vi "Image_Crop_Fixed_Area_old.vi"(8 "Particle Measurements":dbl[][](array[numeric]), 9 "Image":T1, 11 "Object size threshold":dbl=500.0) -> (0 "Object detected":bool, 3 "output array":i32[](array[numeric]))   [LabVIEW 2019]
uses:
  <vilib>/vision/Image Controls.llb/IMAQ Image.ctl
panel:
  out "error out":errorcluster={"status"=TRUE, "code"=-1074396120, "source"="IMAQ Get Image Size\n  "}
  out "Image size/2":dbl
  out "Max x":dbl
  out "Max y":dbl
  in  "Image Border":dbl=20.0
  out "Max area detected":dbl
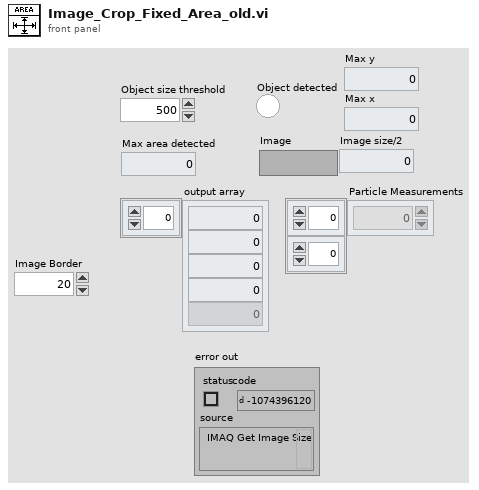
[diagram p1: front panel]
types:
  T1 = typedef "IMAQ Image.ctl" = refnum<image>
  T2 = cluster{"Global Rectangle":i32[], "Contours":cluster{"ID":enum32{"External", "Internal"}, "Type":u32, "Coordinates":i32[]}[]}
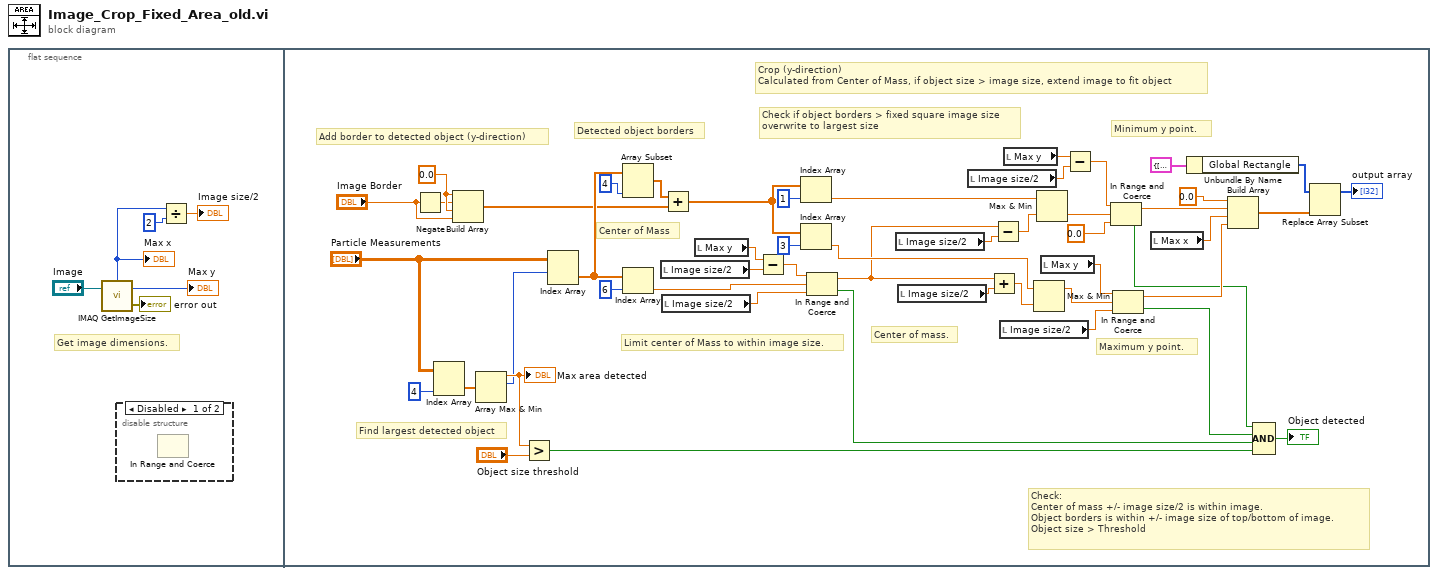
[diagram p0: block diagram]
diagram:
  n1 = flat-sequence {
    frame #0 {
      # "Get image dimensions."
      n2 = call "IMAQ GetImageSize"("Image"="Image") -> ("Y Resolution"=→"Max y":i32, "X Resolution"=w4:i32, "error out"=→"error out":errorcluster)  [unwired: 3 in]
      "Max x" <- w4
      n3 = disable-structure shown="Disabled" {
        frame Disabled {
          n4 = In Range and Coerce() -> ()  [unwired: 3 in, 2 out]
        }
        frame Enabled {
        }
      }
      n5 = Divide(x=w4, y=2) -> (x/y=→"Image size/2":dbl)
    }
    frame #1 {
      w39 = 0.0 ("element")
      # "Check:\nCenter of mass +/- image size/2 is within image.\nObject borders is within +/- image size of top/bottom of image.\nObject size > Threshold"
      # "Maximum y point."
      # "Minimum y point."
      # "Center of mass."
      # "Limit center of Mass to within image size."
      # "Add border to detected object (y-direction)"
      # "Find largest detected object"
      # "Check if object borders > fixed square image size\noverwrite to largest size"
      # "Detected object borders"
      # "Center of Mass"
      # "Crop (y-direction)\nCalculated from Center of Mass, if object size > image size, extend image to fit object"
      n6 = Negate(x="Image Border") -> (-x=w37:dbl)
      n7 = Index Array(array="Particle Measurements", index (col)=4 ("index (row)")) -> (element=w52:dbl[])  [unwired: 1 in]
      n8 = Build Array(w39, w37, w39, "Image Border") -> (w36:dbl[])
      n9 = Array Max & Min(array=w52) -> (max value=w50:dbl, max index (indices)=w47:i32)  [unwired: 2 out]
      "Max area detected" <- w50
      n10 = Greater?(x=w50, y="Object size threshold") -> (0:w49:bool)
      n11 = Index Array(array="Particle Measurements", index (row)=w47) -> (element=w46:dbl[])  [unwired: 1 in]
      n12 = Array Subset(array=w46, length=4) -> (w44:dbl[])  [unwired: 1 in]
      n13 = Index Array(array=w46, index=6) -> (element=w24:dbl)
      n14 = local read "Image size/2"() -> (w30:dbl)
      n15 = local read "Image size/2"() -> (w22:dbl)
      n16 = Add(x=w44, y=w36) -> (x+y=w27:dbl[])
      n17 = local read "Max y"() -> (w31:dbl)
      n18 = Subtract(x=w31, y=w30) -> (x-y=w23:dbl)
      n19 = Index Array(array=w27, index=1) -> (element=w42:dbl)
      n20 = Index Array(array=w27, index=3) -> (element=w40:dbl)
      n21 = In Range and Coerce(upper limit=w23, x=w24, lower limit=w22) -> (coerced(x)=w20:dbl, In Range?=w21:bool)
      n22 = local read "Image size/2"() -> (w26:dbl)
      n23 = local read "Image size/2"() -> (w25:dbl)
      n24 = local read "Image size/2"() -> (w15:dbl)
      n25 = Add(x=w20, y=w25) -> (x+y=w29:dbl)
      n26 = Subtract(x=w20, y=w26) -> (x-y=w28:dbl)
      n27 = local read "Image size/2"() -> (w12:dbl)
      n28 = local read "Max y"() -> (w16:dbl)
      n29 = Max & Min(x=w40, y=w29) -> (max(x,y)=w7:dbl)  [unwired: 1 out]
      n30 = Max & Min(x=w42, y=w28) -> (min(x,y)=w19:dbl)  [unwired: 1 out]
      n31 = local read "Max y"() -> (w13:dbl)
      n32 = Subtract(x=w16, y=w15) -> (x-y=w14:dbl)
      n33 = In Range and Coerce(upper limit=w14, x=w19, lower limit=0.0 ("x")) -> (coerced(x)=w17:dbl, In Range?=w9:bool)
      n34 = In Range and Coerce(upper limit=w13, x=w7, lower limit=w12) -> (coerced(x)=w11:dbl, In Range?=w10:bool)
      n35 = local read "Max x"() -> (w32:dbl)
      n36 = Unbundle By Name(T2 {"Global Rectangle"=[106, 29, 356, 265], "Contours"=[{"ID"=enum."External", "Type"=3, "Coordinates"=[106, 29, 356, 265]}]} ("Crop to object")) -> ("Global Rectangle"=w55:i32[])
      n37 = Build Array(0.0 ("x"), w17, w32, w11) -> (w35:dbl[])
      n38 = Compound Arithmetic op=AND(w9, w10, w21, w49) -> (→"Object detected":bool)
      n39 = Replace Array Subset(array=w55, new element=w35) -> (→"output array":i32[])  [unwired: 1 in]
    }
  }
